vi "dec2bin.vi"(1 "Decimal Input":u8[](array[numeric])) -> (0 "Logical output":bool[](array[boolean]))   [LabVIEW 2019]
uses:
  D:/TFS-Labview/NI 2019/TCSS_V1.0-2021.10.18/TCSS/TCSS/TCSS Project/icon/Down.ctl
  D:/TFS-Labview/NI 2019/TCSS_V1.0-2021.10.18/TCSS/TCSS/TCSS Project/icon/Up.ctl
panel:
  out "Pressure Inside 1703":T3
  out "Binary Output":i16[](array[numeric])
  # "Pad 1"
  # "Pad 2"
  # "Pad 3"
  # "Pad 4"
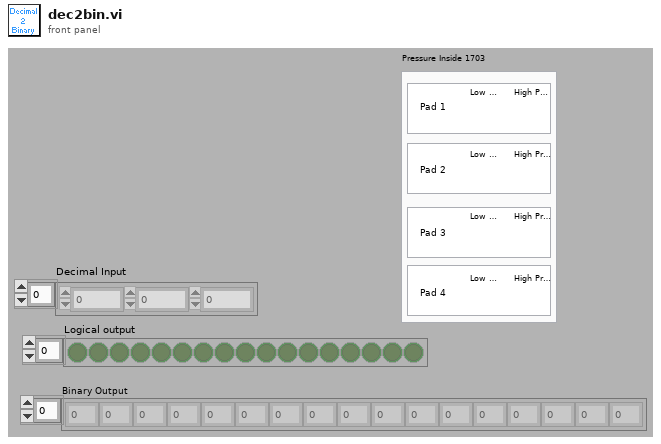
[diagram p1: front panel]
types:
  T1 = typedef "Down.ctl" = u16
  T2 = typedef "Up.ctl" = u16
  T3 = cluster{"Low Pressure":T1, "High Pressure":T2, "Low Pressure":T1, "High Pressure":T2, "Low Pressure":T1, "High Pressure":T2, "Low Pressure":T1, "High Pressure":T2}
  T4 = cluster{"[0]":i16, "[1]":i16, "[2]":i16, "[3]":i16, "[4]":i16, "[5]":i16, "[6]":i16, "[7]":i16}
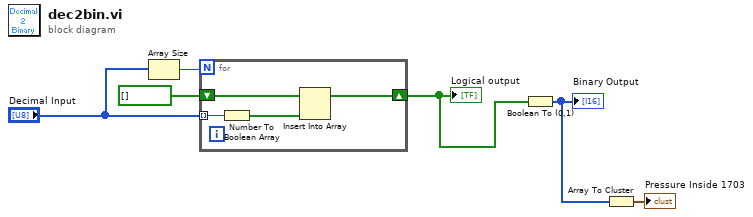
[diagram p0: block diagram]
diagram:
  n1 = Array Size(array="Decimal Input") -> (size(s)=w5:i32)
  n2 = for {
    N: w5 -> [_]
    tunnel: "Decimal Input" -> [w10] mode=indexing
    shift-right: [w8] -> w3
    shift-left: bool[] [] ("array") -> [w9]
    n3 = Number To Boolean Array(number=w10) -> (Boolean array=w7:bool[])
    n4 = Insert Into Array(array=w9, new element=w7) -> (w8:bool[])  [unwired: 1 in]
  }
  "Logical output" <- w3
  n5 = Boolean To (0,1)(Boolean=w3) -> (0, 1=w1:i16[])
  "Binary Output" <- w1
  n6 = Array To Cluster(array=w1) -> (cluster=→"Pressure Inside 1703":T4)
